vi "Ammeter.vi"(9 "Bor - Frequency [Hz]":dbl, 10 "Måling ammeter":dbl, 11 "Sum batteri shift in":dbl) -> (1 "Wait ud":dbl, 2 "Sum batteri shift ud":dbl, 3 "Batteri tilbage (%)":dbl, 4 "Målt ampere":dbl)   [LabVIEW 2019]
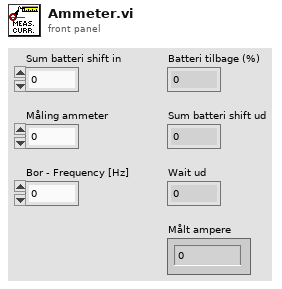
[diagram p1: front panel]
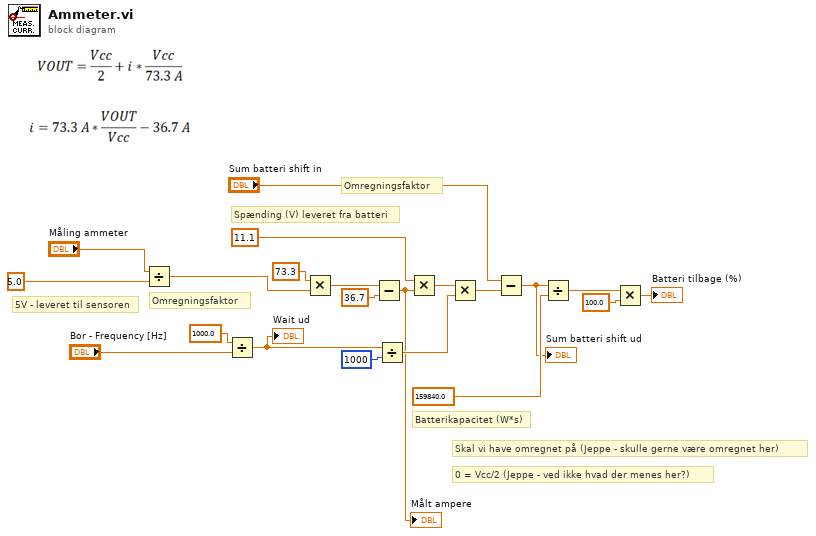
[diagram p0: block diagram]
diagram:
  # "Batterikapacitet (W*s)"
  # "Spænding (V) leveret fra batteri"
  # "Omregningsfaktor"
  # "Omregningsfaktor"
  # "5V - leveret til sensoren"
  # "Skal vi have omregnet på (Jeppe - skulle gerne være omregnet her)"
  # "0 = Vcc/2 (Jeppe - ved ikke hvad der menes her?)"
  n1 = Divide(x="Måling ammeter", y=5.0) -> (x/y=w4:dbl)
  n2 = Divide(x=1000.0, y="Bor - Frequency [Hz]") -> (x/y=w21:dbl)
  "Wait ud" <- w21
  n3 = Multiply(x=73.3, y=w4) -> (x*y=w6:dbl)
  n4 = Subtract(x=w6, y=36.7) -> (x-y=w9:dbl)
  "Målt ampere" <- w9
  n5 = Divide(x=w21, y=u32 1000) -> (x/y=w12:dbl)
  n6 = Multiply(x=11.1, y=w9) -> (x*y=w10:dbl)
  n7 = Multiply(x=w10, y=w12) -> (x*y=w13:dbl)
  n8 = Subtract(x="Sum batteri shift in", y=w13) -> (x-y=w15:dbl)
  "Sum batteri shift ud" <- w15
  n9 = Divide(x=w15, y=159840.0) -> (x/y=w17:dbl)
  n10 = Multiply(x=w17, y=100.0) -> (x*y=→"Batteri tilbage (%)":dbl)
